vi "SetBDAT.vi"(8 "error in (no error)":errorcluster) -> (0 "error out":errorcluster)   [LabVIEW 2015, in "ESLSCDLL.lvlib"]
uses:
  ESLSCDLL.lvlib
  Globals.vi
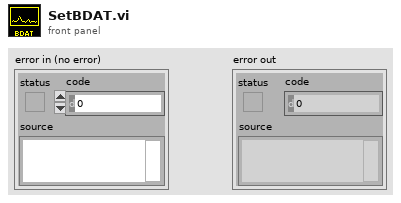
[diagram p1: front panel]
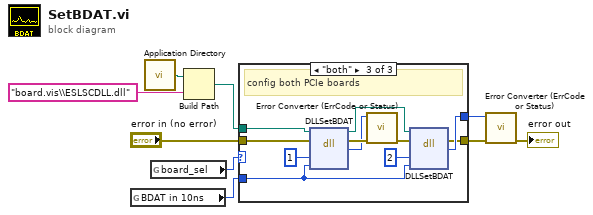
[diagram p0: block diagram]
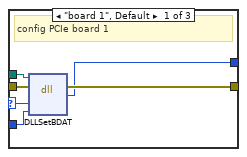
[diagram p2: hidden frame]
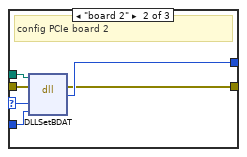
[diagram p3: hidden frame]
diagram:
  n1 = global read "Globals.vi" "BDAT in 10ns"() -> (w4:u32)
  n2 = call <vilib>:"Application Directory.vi"() -> ("Application Directory"=w3:path)
  n3 = global read "Globals.vi" "board_sel"() -> (w5:enum32{"0", "board 1", "board 2", "both"})
  n4 = Build Path(base path=w3, name or relative path="board.vis\\ESLSCDLL.dll") -> (appended path=w1:path)
  n5 = case shown="\"both\"" w5 {
    selector: w5 -> [w15 w20 _]
    tunnel: "error in (no error)" -> [w14 w21 w32]
    tunnel: [w13 w17 w26] -> w8
    tunnel: [w12 w18 w27] -> w6
    tunnel: w4 -> [w11 w19 w28]
    tunnel: w1 -> [w10 w16 w23]
    frame "board 1", Default {
      # "config PCIe board 1"
      n6 = dll-call lib="C:/ENTW/PCIE/LV64/board.vis/ESLSCDLL.dll" fn="DLLSetBDAT" ("lwlscdll.dll:DLLSetTemp")(path in=w10, error in=w14, "drv"=w15, "bdat_in_100ns"=w11) -> (error out=w13:errorcluster, "es_status_codes"=w12:i32)  [unwired: 3 in, 1 out]
    }
    frame "board 2" {
      # "config PCIe board 2"
      n7 = dll-call lib="C:/ENTW/PCIE/LV64/board.vis/ESLSCDLL.dll" fn="DLLSetBDAT" ("lwlscdll.dll:DLLSetTemp")(path in=w16, error in=w21, "drv"=w20, "bdat_in_100ns"=w19) -> (error out=w17:errorcluster, "es_status_codes"=w18:i32)  [unwired: 3 in, 1 out]
    }
    frame "both" {
      # "config both PCIe boards"
      n8 = dll-call lib="C:/ENTW/PCIE/LV64/board.vis/ESLSCDLL.dll" fn="DLLSetBDAT" ("lwlscdll.dll:DLLSetTemp")(path in=w23, error in=w32, "drv"=u32 1, "bdat_in_100ns"=w28) -> (path out=w22:path, error out=w25:errorcluster, "es_status_codes"=w24:i32)  [unwired: 3 in]
      n9 = call "Error Converter (ErrCode or Status).vi"("error in (no error)"=w25, "error code"=w24) -> ("error out"=w30:errorcluster)  [unwired: 9 in]
      n10 = dll-call lib="C:/ENTW/PCIE/LV64/board.vis/ESLSCDLL.dll" fn="DLLSetBDAT" ("lwlscdll.dll:DLLSetTemp")(path in=w22, error in=w30, "drv"=u32 2, "bdat_in_100ns"=w28) -> (error out=w26:errorcluster, "es_status_codes"=w27:i32)  [unwired: 3 in, 1 out]
    }
  }
  n11 = call "Error Converter (ErrCode or Status).vi"("error in (no error)"=w8, "error code"=w6) -> ("error out"=→"error out":errorcluster)  [unwired: 9 in]
